vi "Check Interlock.vi"(8 "Error In":errorcluster, 10 "Water Pressure Sensor (%)":u32, 11 "Rain Sensor":bool) -> (0 "Error Out":errorcluster, 2 "State In":string, 3 "Water Ok?":bool)   [LabVIEW 2024]
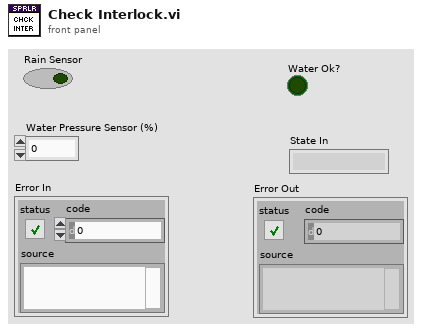
[diagram p1: front panel]
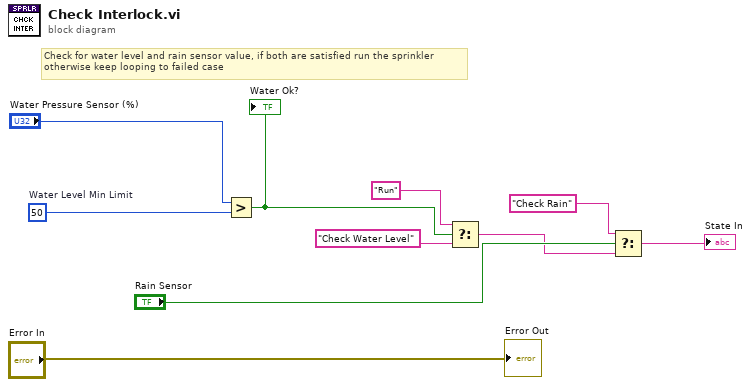
[diagram p0: block diagram]
diagram:
  w6 = u32 50  # Water Level Min Limit
  # "Check for water level and rain sensor value, if both are satisfied run the sprinkler \notherwise keep looping to failed case"
  n1 = Greater?(x="Water Pressure Sensor (%)", y=w6) -> (0:w10:bool)
  "Water Ok?" <- w10
  n2 = Select(t="Run" ("State In"), s=w10, f="Check Water Level" ("State In")) -> (s? t:f=w1:string)
  n3 = Select(t="Check Rain" ("State In"), s="Rain Sensor", f=w1) -> (s? t:f=→"State In":string)
  "Error Out" <- "Error In"
